vi "Get Raw Data.vi"(7 "Use Cached Data?":bool, 8 "Error In":errorcluster, 11 "Nest Config":T1) -> (0 "Error Out":errorcluster, 1 "Data":string, 3 "Nest Config":T1)   [LabVIEW 2013, in "LMH-Nest.lvlib"]
doc: "Get all Nest data. By default this VI queries the Nest server. Set Use Chaced Data? to true to used the chaced data to avoid pinging the Nest server."
uses:
  LMH-Nest.lvlib
  Type Defs/Nest Config.ctl
  <vilib>/httpClient/ClientHandle.ctl
  Type Defs/Session Data.ctl
  Type Defs/Nest Data FGV State.ctl
  Type Defs/Nest Error.ctl
  <vilib>/httpClient/LabVIEWHTTPClient.lvlib
  <vilib>/express/express shared/NI_ExcelFile/NI_ExcelFile.lvlib
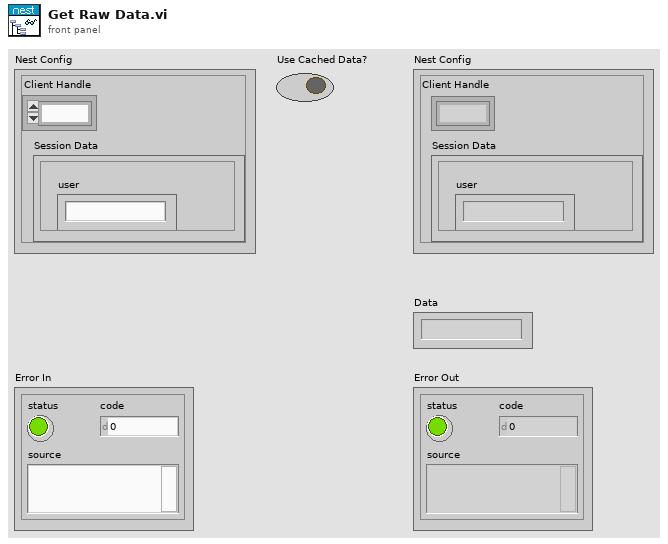
[diagram p1: front panel]
types:
  T1 = typedef "LMH-Nest.lvlib/Nest Config.ctl" = cluster{"Client Handle":T2, "Session Data":T3}
  T2 = typedef "LabVIEWHTTPClient.lvlib/ClientHandle.ctl" = refnum<k1>
  T3 = typedef "LMH-Nest.lvlib/Session Data.ctl" = cluster{"is_superuser":bool, "is_staff":bool, "urls":cluster{"transport_url":string, "rubyapi_url":string, "weather_url":string, "log_upload_url":string, "support_url":string}, "limits":cluster{"thermostats_per_structure":u32, "structures":u32, "thermostats":u32, "smoke_detectors":u32, "smoke_detectors_per_structure":u32}, "access_token":string, "userid":string, "expires_in":string, "email":string, "user":string, "language":string}
  T4 = typedef "LMH-Nest.lvlib/Nest Data FGV State.ctl" = enum16{"Init", "Set", "Get"}
  T5 = typedef "LMH-Nest.lvlib/Nest Error.ctl" = enum16{"Unknown", "Auth", "Read", "Invalid Structure Name", "Invalid Device Name", "Set Temp"}
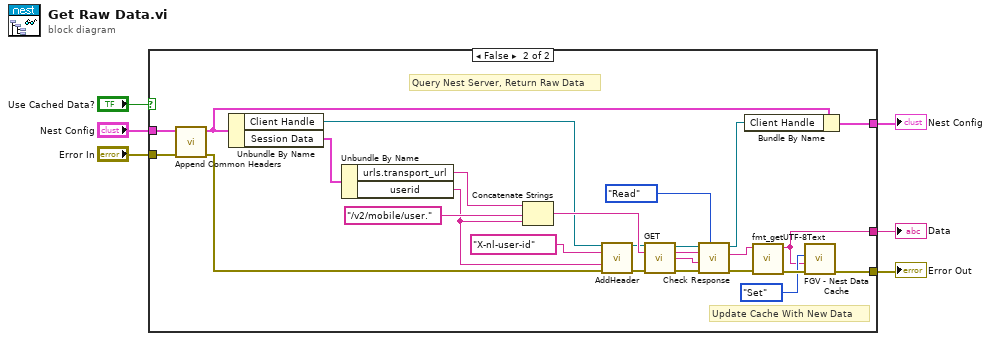
[diagram p0: block diagram]
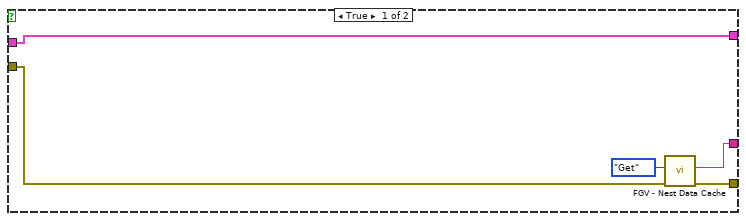
[diagram p2: hidden frame]
diagram:
  n1 = case shown="False" "Use Cached Data?" {
    tunnel: "Nest Config" -> [w7 w30]
    tunnel: "Error In" -> [w10 w29]
    tunnel: [w7 w24] -> w4
    tunnel: [w8 w12] -> w3
    tunnel: [w11 w14] -> w2
    frame True {
      n2 = call "FGV - Nest Data Cache.vi"("Error In"=w10, "Nest Data FGV State"=Nest_Data_FGV_State."Get") -> ("Error Out"=w11:errorcluster, "Nest Cached Data"=w8:string)  [unwired: 8 in]
    }
    frame False {
      # "Update Cache With New Data"
      # "Query Nest Server, Return Raw Data"
      n3 = call "Append Common Headers.vi"("Error In"=w29, "Nest Config"=w30) -> ("Error Out"=w26:errorcluster, "Nest Config"=w25:T1)  [unwired: 8 in]
      n4 = Unbundle By Name(w25) -> ("Client Handle"=w27:T2, "Session Data"=w28:T3)
      n5 = Unbundle By Name(w28) -> ("urls.transport_url"=w37:string, "userid"=w33:string)
      n6 = Concatenate Strings(w37, "/v2/mobile/user.", w33) -> (w34:string)
      n7 = call <vilib>:"AddHeader.vi"("client handle"=w27, "header"="X-nl-user-id", "value"=w33, "error in (no error)"=w26) -> ("client handle out"=w31:T2, "error out"=w32:errorcluster)  [unwired: 10 in]
      n8 = call <vilib>:"GET.vi"("client handle"=w31, "url"=w34, "error in (no error)"=w32) -> ("client handle out"=w20:T2, "headers"=w21:string, "body"=w22:string, "error out"=w23:errorcluster)  [unwired: 9 in]
      n9 = call "Check Response.vi"("Nest Error"=Nest_Error."Read", "Error In"=w23, "Body"=w22, "Header"=w21, "Client Handle"=w20) -> ("Error Out"=w16:errorcluster, "Body"=w17:string, "Client Handle"=w19:T2)  [unwired: 3 in, 1 out]
      n10 = Bundle By Name(cluster=w25, "Client Handle"=w19) -> (w24:T1)
      n11 = call <vilib>:"fmt_getUTF-8Text.vi"("error in"=w16, "plain text"=w17) -> ("error out"=w15:errorcluster, "utf-8 text"=w12:string)  [unwired: 8 in]
      n12 = call "FGV - Nest Data Cache.vi"("Error In"=w15, "Nest Data"=w12, "Nest Data FGV State"=Nest_Data_FGV_State."Set") -> ("Error Out"=w14:errorcluster)  [unwired: 7 in, 1 out]
    }
  }
  "Error Out" <- w2
  "Nest Config" <- w4
  "Data" <- w3
